vi "Build String plus underscore.vi"(6 "Append Extension":bool, 7 "Separator charactor":string, 8 "Append":string, 11 "Input String":string) -> (3 "Output String":string)   [LabVIEW 2017]
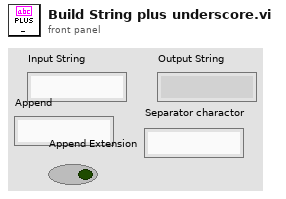
[diagram p1: front panel]
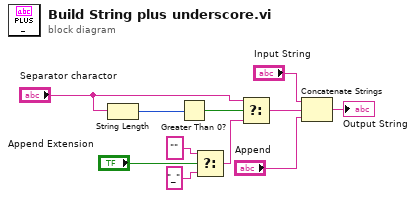
[diagram p0: block diagram]
diagram:
  n1 = String Length(string="Separator charactor") -> (length=w8:i32)
  n2 = Greater Than 0?(x=w8) -> (x > 0?=w7:bool)
  n3 = Select(t="", s="Append Extension", f="_") -> (s? t:f=w1:string)
  n4 = Select(t="Separator charactor", s=w7, f=w1) -> (s? t:f=w6:string)
  n5 = Concatenate Strings("Input String", w6, "Append") -> (→"Output String":string)
